vi "OAT Reshape Resample Result.vi"(10 "channel count":i32=1, 11 "output":dbl[](array[numeric]) format="%.2f") -> (2 "output len":i32, 3 "Y":dbl[][](array[numeric]) format="%.2f")   [LabVIEW 2017, in "SoundVib_Resampling.lvlib"]
uses:
  <vilib>/addons/Sound and Vibration/Order Analysis/Resample Order Tracking/SoundVib_Resampling.lvlib
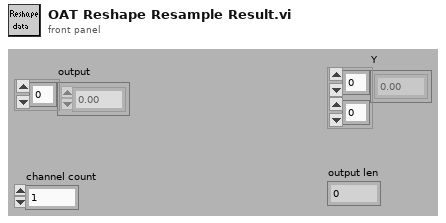
[diagram p1: front panel]
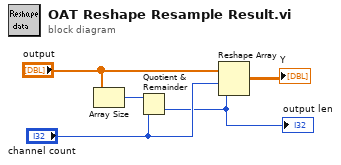
[diagram p0: block diagram]
diagram:
  n1 = Array Size(array="output") -> (size(s)=w5:i32)
  n2 = Quotient & Remainder(x=w5, y="channel count") -> (floor(x/y)=w2:i32)  [unwired: 1 out]
  "output len" <- w2
  n3 = Reshape Array("output", "channel count", w2) -> (→"Y":dbl[][])
